vi "Create-Window.vi"(8 "error in (no error)":errorcluster) -> (0 "error out":errorcluster, 3 "Window":refnum<class "Window.lvclass">)   [LabVIEW 2020, in "GLF.lvlib" / "Window.lvclass"]
uses:
  Window.lvclass
  Window.lvclass/Window.ctl
  Engine/Engine.lvclass
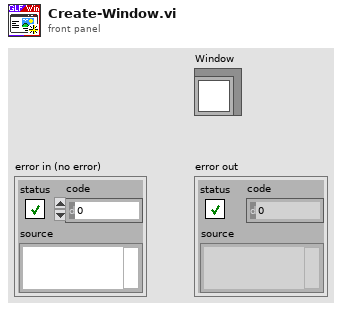
[diagram p1: front panel]
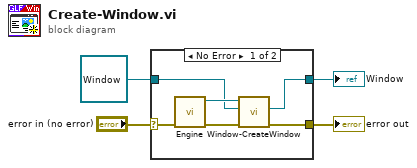
[diagram p0: block diagram]
diagram:
  n1 = case shown="No Error" "error in (no error)" {
    selector: "error in (no error)" -> [w9 w12]
    tunnel: [w7 w12] -> w3
    tunnel: [w5 w11] -> w1
    tunnel: refnum<class "Window.lvclass"> refnum ("Window in") -> [w6 w11]
    frame No Error {
      n2 = call "Engine.vi"("error in (no error)"=w9) -> ("error out"=w8:errorcluster, "Engine"=w10:refnum<class "Engine.lvclass">)  [unwired: 9 in]
      n3 = call "Window-CreateWindow.vi"("error in (no error)"=w8, "Window Type"=w6, "Engine in"=w10) -> ("error out"=w7:errorcluster, "Window Instance"=w5:refnum<class "Window.lvclass">)  [unwired: 6 in, 1 out]
    }
    frame Error {
    }
  }
  "error out" <- w3
  "Window" <- w1
